vi "Wait Event Callback.vi"(4 "Top level VI":refnum<vi>, 5 "Event data":cluster{"showWait":bool}, 6 "CtlRef":refnum<k7>, 7 "Event common data":cluster{"Source":i32, "Type":u32, "Time":u32}) -> ()   [LabVIEW 2025]
doc: "The Application Manager generates the Wait event at the beginning and end of\nlengthy operations. The operator interface can then display a wait cursor to\nindicate to the user that the operator interface is busy."
uses:
  <vilib>/Utility/cursorutil.llb/Set Cursor (Icon Pict).vi
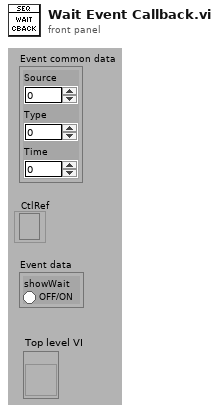
[diagram p1: front panel]
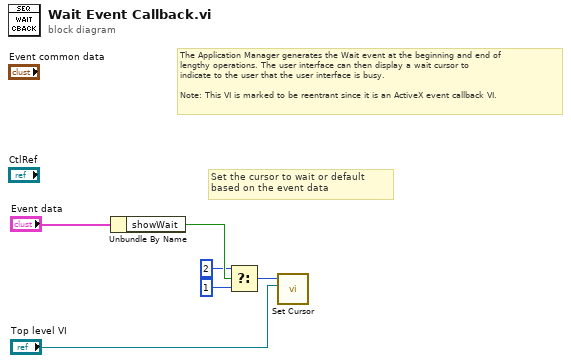
[diagram p0: block diagram]
diagram:
  # "Set the cursor to wait or default based on the event data"
  # "The Application Manager generates the Wait event at the beginning and end of\nlengthy operations. The user interface can then display a wait cursor to\nindicate to the user that the user interface is busy.\n\nNote: This VI is marked to be reentrant since it is an ActiveX event callback VI."
  n1 = Unbundle By Name("Event data") -> ("showWait"=w4:bool)
  n2 = Select(t=u16 2 ("icon"), s=w4, f=u16 1 ("icon")) -> (s? t:f=w2:u16)
  n3 = call-poly <vilib>:"Set Cursor.vi"("VI reference (current VI)"="Top level VI", "icon"=w2) -> ()  [unwired: 8 in, 2 out]
